vi "Make snp from MDIF file.vi"() -> ()   [LabVIEW 2020]
panel:
  in  "Var index offset":i32
  in  "File name format":string="WS-EVB-225b 3778A (%d)_DUT.s2p"
  out "error out":errorcluster
  in  "file (use dialog)":path
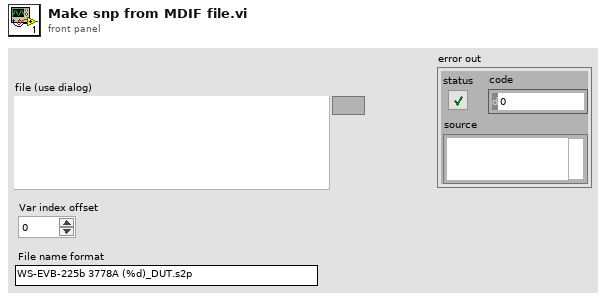
[diagram p1: front panel]
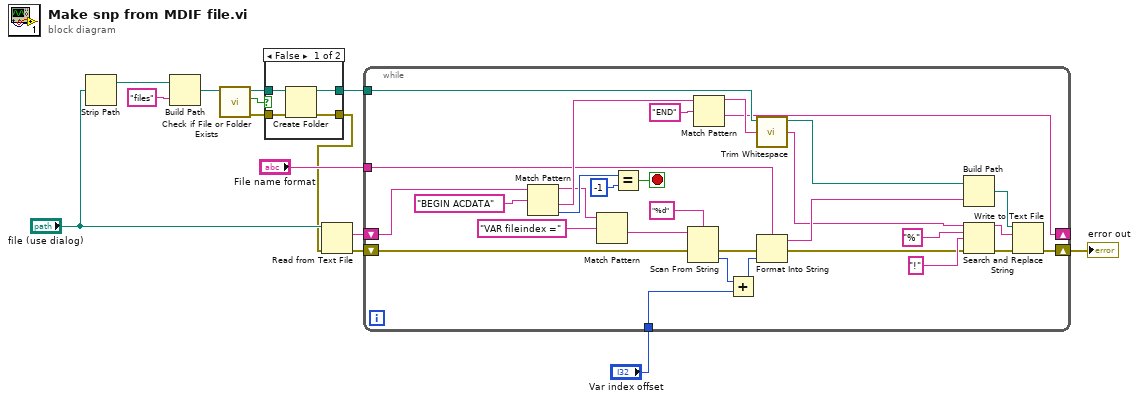
[diagram p0: block diagram]
diagram:
  n1 = Strip Path(path="file (use dialog)") -> (stripped path=w12:path)  [unwired: 1 out]
  n2 = Build Path(base path=w12, name or relative path="files") -> (appended path=w7:path)
  n3 = call <vilib>:"Check if File or Folder Exists.vi"("path"=w7) -> ("error out"=w4:errorcluster, "file or folder exists?"=w6:bool, "dup path"=w5:path)  [unwired: 8 in]
  n4 = case shown="False" w6 {
    tunnel: w5 -> [w18 w20]
    tunnel: w4 -> [w17 w19]
    tunnel: [w16 w20] -> w3
    tunnel: [w15 w19] -> w2
    frame False {
      n5 = Create Folder(path (use dialog)=w18, error in=w17) -> (created path=w16:path, error out=w15:errorcluster)  [unwired: 1 in, 1 out]
    }
    frame True {
    }
  }
  n6 = Read from Text File(file (use dialog)="file (use dialog)", error in=w2) -> (text=w14:string, error out=w10:errorcluster)  [unwired: 2 in, 2 out]
  n7 = while {
    shift-right: [w34] -> _
    shift-left: w14 -> [w49]
    tunnel: w3 -> [w43]
    shift-right: [w25] -> w9
    shift-left: w10 -> [w26]
    tunnel: "File name format" -> [w24]
    tunnel: "Var index offset" -> [w21]
    stop <- w44 stop-if-true
    n8 = Match Pattern(string=w49, regular expression="BEGIN ACDATA") -> (before substring=w38:string, after substring=w40:string, offset past match=w45:i32)  [unwired: 1 in, 1 out]
    n9 = Match Pattern(string=w38, regular expression="VAR fileindex =") -> (after substring=w36:string)  [unwired: 1 in, 3 out]
    n10 = Equal?(x=w45, y=-1 ("offset past match")) -> (x = y?=w44:bool)
    n11 = Scan From String(format string="%d" ("regular expression"), input string=w36, error in=w26) -> (error out=w27:errorcluster, output 1=w23:i32)  [unwired: 2 in, 2 out]
    n12 = Match Pattern(string=w40, regular expression="END") -> (before substring=w35:string, after substring=w34:string)  [unwired: 1 in, 2 out]
    n13 = Add(x=w23, y=w21) -> (x+y=w22:i32)
    n14 = call <vilib>:"Trim Whitespace.vi"("string"=w35) -> ("trimmed string"=w33:string)  [unwired: 1 in]
    n15 = Format Into String(format string=w24, error in=w27, w22) -> (resulting string=w42:string, error out=w28:errorcluster)  [unwired: 1 in]
    n16 = Build Path(base path=w43, name or relative path=w42) -> (appended path=w39:path)
    n17 = Search and Replace String(input string=w33, search string="%", replace string="!" ("replace string (\"\")"), error in=w28) -> (result string=w32:string, error out=w29:errorcluster)  [unwired: 4 in, 2 out]
    n18 = Write to Text File(file (use dialog)=w39, text=w32, error in=w29) -> (error out=w25:errorcluster)  [unwired: 1 in, 2 out]
  }
  "error out" <- w9
